vi "国弘测量偏移修正值.vi"(7 "探头":u16(ring)=5 items=["NULL", "pH", "Cond", "DO", "Turb", "ORP", "6", "7", "8", "9", "氯化物"], 8 "error in (no error)":errorcluster caption="错误输入（无错误）", 11 "温度偏移修正值":sgl) -> (0 "error out":errorcluster caption="错误输出", 3 "MB session out":refnum<class "MB_Master.lvclass">)   [LabVIEW 2016, in "斯坦道多参数.lvlib"]
uses:
  <vilib>/Plasmionique/MB Master/MB_Master/MB_Master.lvclass
  <vilib>/Plasmionique/MB Master/MB Master.lvlib
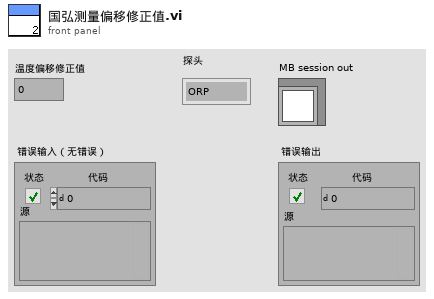
[diagram p1: front panel]
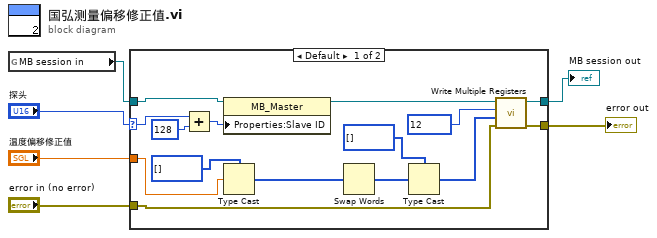
[diagram p0: block diagram]
diagram:
  n1 = global read "多参数全局变量.vi" "MB session in"() -> (w1:refnum<class "MB_Master.lvclass">)
  n2 = case shown="Default" "探头" {
    selector: "探头" -> [w7 _]
    tunnel: "error in (no error)" -> [w20 w22]
    tunnel: "温度偏移修正值" -> [w12 _]
    tunnel: w1 -> [w10 w23]
    tunnel: [w9 w22] -> w4
    tunnel: [w8 w23] -> w3
    frame Default {
      n3 = Add(x=w7, y=u16 128) -> (x+y=w19:u16)
      n4 = property class="MB_Master"(reference=w10, "Properties:Slave ID"=w19) -> (reference out=w17:refnum<class "MB_Master.lvclass">)  [unwired: 1 in, 1 out]
      n5 = Type Cast(type=u32[] [] ("数组 2"), x=w12) -> (*(type *) &x=w15:u32[])
      n6 = Swap Words(1:w15) -> (0:w13:u32[])
      n7 = Type Cast(type=u16[] [] ("数组 2"), x=w13) -> (*(type *) &x=w11:u16[])
      n8 = call <vilib>:"Write Multiple Registers.vi"("error in (no error)"=w20, "values"=w11, "starting address"=u16 12, "MB session in"=w17) -> ("error out"=w9:errorcluster, "MB session out"=w8:refnum<class "MB_Master.lvclass">)  [unwired: 6 in]
    }
    frame 0 {
    }
  }
  "error out" <- w4
  "MB session out" <- w3
